vi "Get Offset Values.vi"(11 "AllOffsetValues":string) -> (3 "OffsetValues":T1)   [LabVIEW 2025]
uses:
  Station/Controls/Offset_Values.ctl
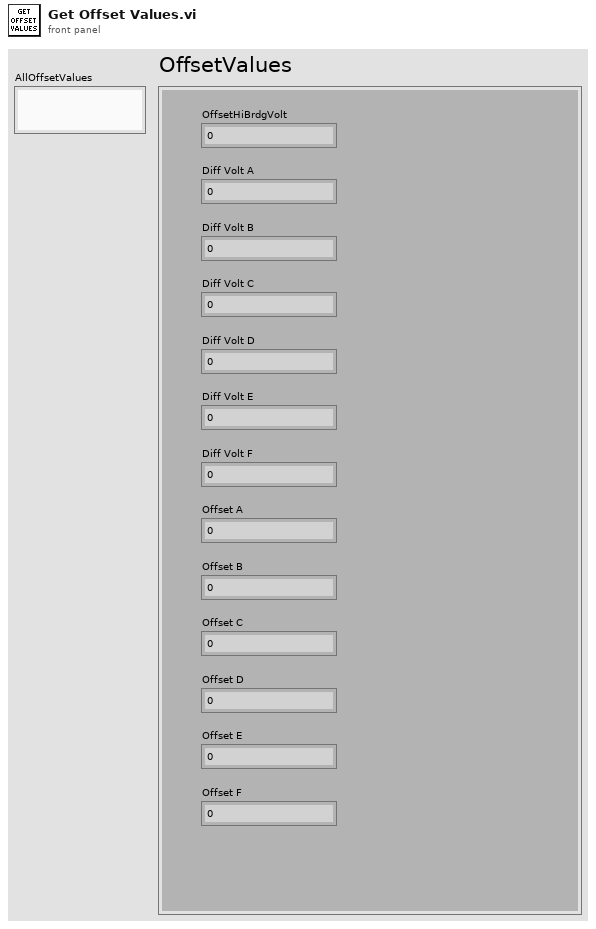
[diagram p1: front panel]
types:
  T1 = typedef "Offset_Values.ctl" = cluster{"OffsetHiBrdgVolt":sgl, "Diff Volt A ":sgl, "Diff Volt B":sgl, "Diff Volt C":sgl, "Diff Volt D":sgl, "Diff Volt E":sgl, "Diff Volt F":sgl, "Offset A":sgl, "Offset B":sgl, "Offset C":sgl, "Offset D":sgl, "Offset E":sgl, "Offset F":sgl}
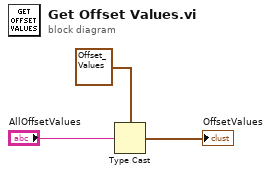
[diagram p0: block diagram]
diagram:
  n1 = Type Cast(type=T1 {"OffsetHiBrdgVolt"=0.0, "Diff Volt A "=0.0, "Diff Volt B"=0.0, "Diff Volt C"=0.0, "Diff Volt D"=0.0, "Diff Volt E"=0.0, "Diff Volt F"=0.0, "Offset A"=0.0, "Offset B"=0.0, "Offset C"=0.0, "Offset D"=0.0, "Offset E"=0.0, "Offset F"=0.0} ("Offset Values"), x="AllOffsetValues") -> (*(type *) &x=→"OffsetValues":T1)
